vi "Session2_Project_Real_Time_Temperature_Display.vi"() -> ()   [LabVIEW 2016]
panel:
  in  "stop":bool
  in  "Sensor Simulator":dbl(slide) scale=0.0..10.0
  in  "Clear":bool
  out "Temp Value":dbl
  out "Thermometer":dbl(slide) scale=0.0..10.0
  out "Temp Chart":dbl(graph)
  # "Session 2 – Project: Real-Time Temperature Display"
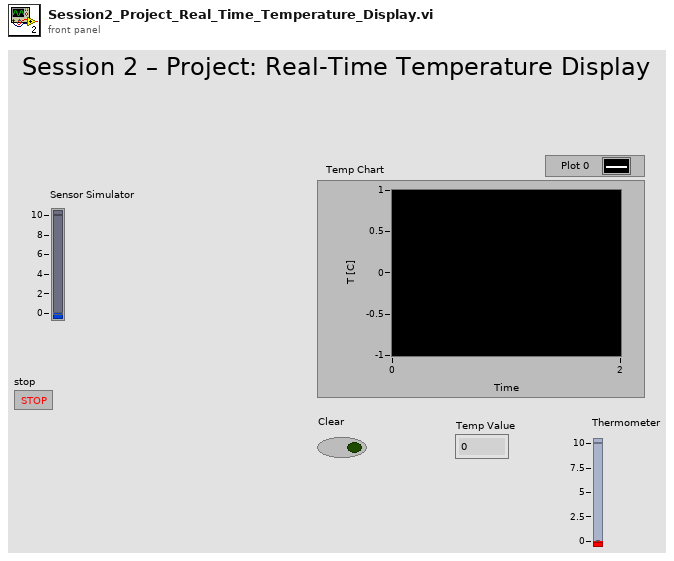
[diagram p1: front panel]
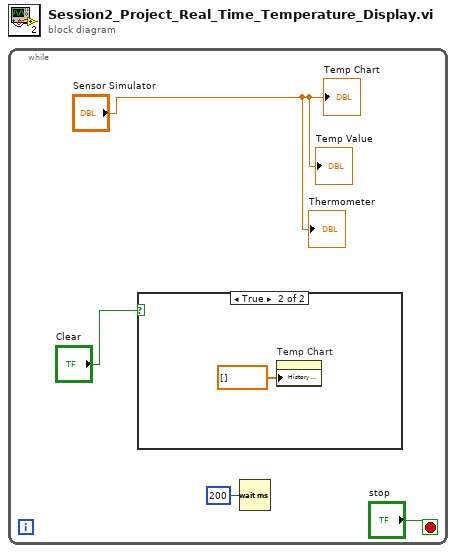
[diagram p0: block diagram]
diagram:
  n1 = while {
    stop <- "stop" stop-if-true
    n2 = case shown="True" "Clear" {
      frame False {
      }
      frame True {
        n3 = property on="Temp Chart" class="WFChart (strict)"("History Data"=dbl[] []) -> ()  [unwired: 2 in, 2 out]
      }
    }
    n4 = Wait (ms)(milliseconds to wait=u32 200) -> ()  [unwired: 1 out]
    "Temp Chart" <- "Sensor Simulator"
    "Temp Value" <- "Sensor Simulator"
    "Thermometer" <- "Sensor Simulator"
  }
